vi "Range Check.vi"(10 "Direction":bool, 11 "Stepper.lvclass":refnum<class "Stepper.lvclass">) -> (1 "Out of range?":bool, 3 "Stepper.lvclass out":refnum<class "Stepper.lvclass">)   [LabVIEW 2009, in "Stepper.lvclass"]
uses:
  Stepper.lvclass
  Stepper.lvclass/Stepper.ctl
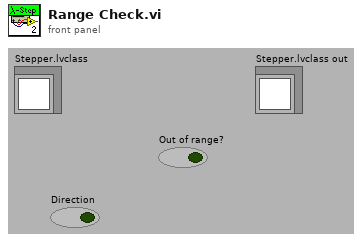
[diagram p1: front panel]
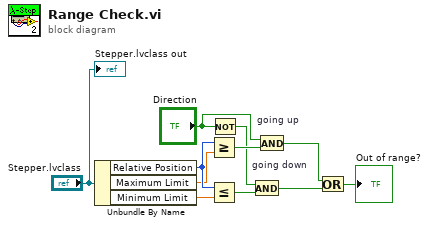
[diagram p0: block diagram]
diagram:
  n1 = Unbundle By Name("Stepper.lvclass") -> ("Relative Position"=w3:i32, "Maximum Limit"=w1:dbl, "Minimum Limit"=w2:dbl)
  n2 = Greater Or Equal?(x=w3, y=w1) -> (x >= y?=w9:bool)
  n3 = Less Or Equal?(x=w3, y=w2) -> (x <= y?=w6:bool)
  n4 = Not(x="Direction") -> (.not. x?=w5:bool)
  n5 = And "going down"(x=w5, y=w6) -> (x .and. y?=w7:bool)
  n6 = And "going up"(x="Direction", y=w9) -> (x .and. y?=w8:bool)
  n7 = Or(x=w8, y=w7) -> (x .or. y?=→"Out of range?":bool)
  "Stepper.lvclass out" <- "Stepper.lvclass"
